vi "Test Sync.vi"() -> ()   [LabVIEW 2019, in "DAQmx.lvclass"]
uses:
  DAQmx.lvclass
  typedefs/DAQ.Config.AO--Cluster--Array.ctl
  typedefs/DAQ.Config.AO--Cluster.ctl
  typedefs/DAQ.Config.AO.Range--enum.ctl
  typedefs/DAQ.Config.Device Type--enum.ctl
  typedefs/DAQ.Config.AI--Cluster--Array.ctl
  typedefs/DAQ.Config.AI--Cluster.ctl
  typedefs/DAQ.Config.AI.Coupling--enum.ctl
  typedefs/DAQ.Config.AI.Range--enum.ctl
  typedefs/DAQ.Config.Timing.Sampling--Cluster.ctl
  typedefs/DAQ.Configuration--Cluster.ctl
  typedefs/DAQ.Config.Timing--Cluster.ctl
  DAQmx.lvclass/DAQmx.ctl
panel:
  out "Numeric":i32
  in  "single device":bool
  in  "Sampling":T1={"Fs"=52000.0, "#s"=5000} {"Fs" format="%#_13g"}
  in  "AI":T2 {"input terminal configuration" items=[""=-1, "Differential"=10106, "Pseudodifferential"=12529]; "Coupling" items=[""=0, "AC"=10045, "DC"=10050, "GND"=10066]}
  in  "AO":T7 {"output terminal configuration" items=[""=-1, "Differential"=10106, "Pseudodifferential"=12529]}
  out "error out":errorcluster
  out "Waveform Graph":waveform(dbl)[](graph)
  in  "stop":bool
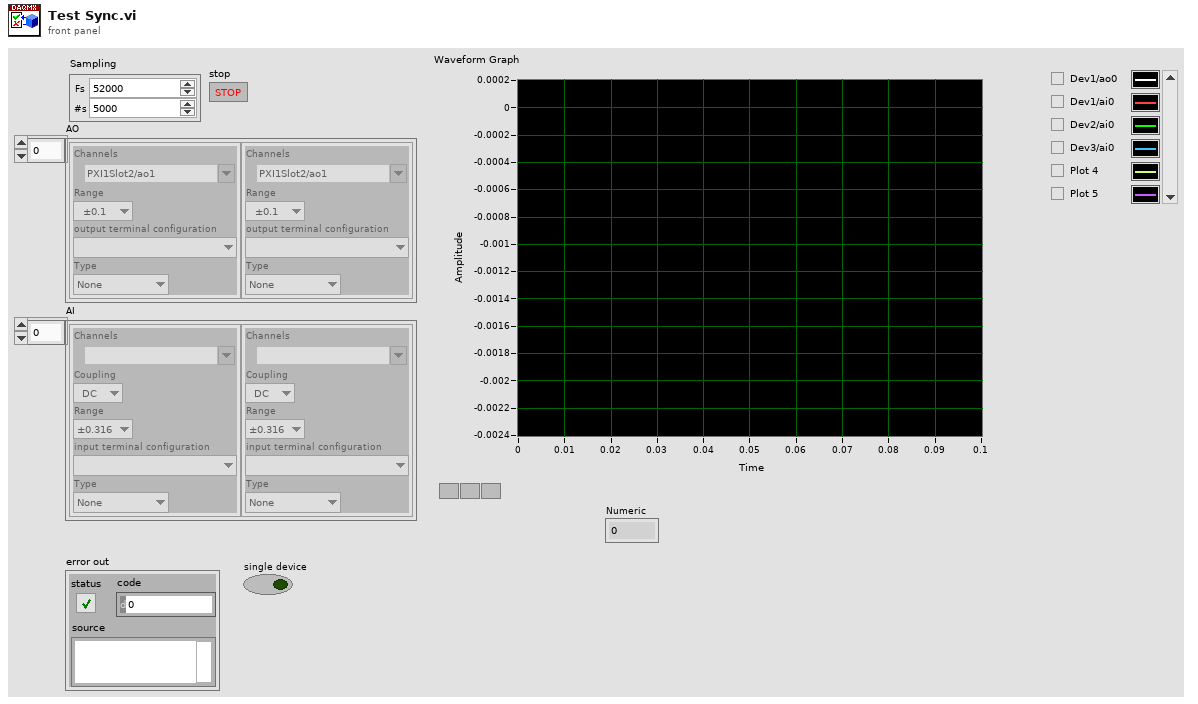
[diagram p1: front panel]
types:
  T1 = typedef "DAQmx.lvclass/DAQ.Config.Timing.Sampling--Cluster.ctl" = cluster{"Fs":dbl, "#s":i32}
  T2 = typedef "DAQmx.lvclass/DAQ.Config.AI--Cluster--Array.ctl" = T3[]
  T3 = typedef "DAQmx.lvclass/DAQ.Config.AI--Cluster.ctl" = cluster{"Channels":tag, "Coupling":T4, "Range":T5, "input terminal configuration":i32, "Type":T6}
  T4 = typedef "DAQmx.lvclass/DAQ.Config.AI.Coupling--enum.ctl" = u16
  T5 = typedef "DAQmx.lvclass/DAQ.Config.AI.Range--enum.ctl" = enum16{"±0.316", "±1.00", "±3.16", "±10.0", "±31.6", "±42.4", ""}
  T6 = typedef "DAQmx.lvclass/DAQ.Config.Device Type--enum.ctl" = enum16{"None", "USB-4431", "PXI-446x"}
  T7 = typedef "DAQmx.lvclass/DAQ.Config.AO--Cluster--Array.ctl" = T8[]
  T8 = typedef "DAQmx.lvclass/DAQ.Config.AO--Cluster.ctl" = cluster{"Channels":tag, "Range":T9, "output terminal configuration":i32, "Type":T6}
  T9 = typedef "DAQmx.lvclass/DAQ.Config.AO.Range--enum.ctl" = enum16{"±0.1", "±1.0", "±3.5", "±10.0", ""}
  T10 = typedef "DAQmx.lvclass/DAQ.Configuration--Cluster.ctl" = cluster{"Timing":T11, "AO":T7, "AI":T2}
  T11 = typedef "DAQmx.lvclass/DAQ.Config.Timing--Cluster.ctl" = cluster{"Sampling":T1, "Fs_Out":dbl}
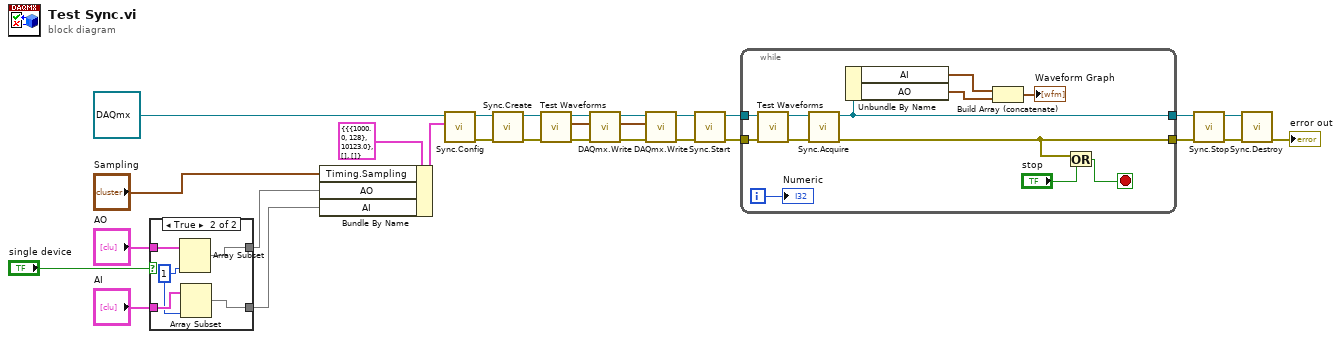
[diagram p0: block diagram]
diagram:
  n1 = case shown="True" "single device" {
    tunnel: [w29 w33] -> w16
    tunnel: "AO" -> [w29 w34]
    tunnel: [w28 w31] -> w14
    tunnel: "AI" -> [w28 w32]
    frame False {
    }
    frame True {
      w30 = 1 ("length")
      n2 = Array Subset(array=w34, length=w30) -> (w33:T7)  [unwired: 1 in]
      n3 = Array Subset(array=w32, length=w30) -> (w31:T2)  [unwired: 1 in]
    }
  }
  n4 = Bundle By Name(cluster=T10 {"Timing"={"Sampling"={"Fs"=1000.0, "#s"=128}, "Fs_Out"=10123.0}, "AO"=[], "AI"=[]} ("Configuration"), "Timing.Sampling"="Sampling", "AO"=w16, "AI"=w14) -> (w11:T10)
  n5 = call "Sync.Config.vi"("Configuration"=w11, "DAQmx in"=refnum<class "DAQmx.lvclass"> refnum) -> ("error out"=w8:errorcluster, "DAQmx out"=w9:refnum<class "DAQmx.lvclass">)  [unwired: 8 in]
  n6 = call "Sync.Create.vi"("error in"=w8, "DAQmx in"=w9) -> ("error out"=w19:errorcluster, "DAQmx out"=w20:refnum<class "DAQmx.lvclass">)  [unwired: 8 in]
  n7 = call "Test Waveforms.vi"("error in (no error)"=w19, "DAQmx in"=w20) -> ("error out"=w4:errorcluster, "Waveforms"=w7:waveform(dbl)[], "DAQmx out"=w5:refnum<class "DAQmx.lvclass">)  [unwired: 7 in]
  n8 = call "DAQmx.Write.vi"("error in (no error)"=w4, "AOwfm"=w7, "DAQmx in"=w5) -> ("error out"=w3:errorcluster, "DAQmx out"=w6:refnum<class "DAQmx.lvclass">)  [unwired: 6 in, 1 out]
  n9 = call "DAQmx.Write.vi"("error in (no error)"=w3, "AOwfm"=w7, "DAQmx in"=w6) -> ("error out"=w2:errorcluster, "DAQmx out"=w1:refnum<class "DAQmx.lvclass">)  [unwired: 6 in, 1 out]
  n10 = call "Sync.Start.vi"("error in"=w2, "DAQmx in"=w1) -> ("error out"=w22:errorcluster, "DAQmx out"=w27:refnum<class "DAQmx.lvclass">)  [unwired: 8 in]
  n11 = while {
    tunnel: w27 -> [w44]
    tunnel: [w39] -> w26
    tunnel: [w42] -> w23
    tunnel: w22 -> [w43]
    i -> [w35]
    stop <- w45 stop-if-true
    n12 = call "Test Waveforms.vi"("error in (no error)"=w43, "DAQmx in"=w44) -> ("error out"=w40:errorcluster, "DAQmx out"=w41:refnum<class "DAQmx.lvclass">)  [unwired: 7 in, 1 out]
    n13 = call "Sync.Acquire.vi"("error in (no error)"=w40, "DAQmx in"=w41) -> ("error out"=w42:errorcluster, "DAQmx out"=w39:refnum<class "DAQmx.lvclass">)  [unwired: 8 in]
    n14 = Unbundle By Name(w39) -> ("AI"=w37:waveform(dbl)[], "AO"=w38:waveform(dbl)[])
    n15 = Build Array (concatenate)(w37, w38) -> (→"Waveform Graph":waveform(dbl)[])
    n16 = Or(x=w42, y="stop") -> (x .or. y?=w45:bool)
    "Numeric" <- w35
  }
  n17 = call "Sync.Stop.vi"("error in (no error)"=w23, "DAQmx in"=w26) -> ("error out"=w24:errorcluster, "DAQmx out"=w25:refnum<class "DAQmx.lvclass">)  [unwired: 8 in]
  n18 = call "Sync.Destroy.vi"("error in (no error)"=w24, "DAQmx in"=w25) -> ("error out"=→"error out":errorcluster)  [unwired: 8 in, 1 out]
